vi "Set Defaults.vi"(11 "Game in":refnum<class "Game.lvclass">) -> (3 "Game out":refnum<class "Game.lvclass">)   [LabVIEW 2020, in "Conditum-Example.lvlib" / "Game.lvclass"]
uses:
  Game.lvclass
  Game.lvclass/Game.ctl
  Conditum/Columns/Entity/Entity.lvclass
  Conditum/Columns/Entity Collection/Entity Collection.lvclass
  Conditum/Columns/String/String.lvclass
  Conditum/Columns/Timestamp/Timestamp.lvclass
  Conditum/Columns/Boolean/Boolean.lvclass
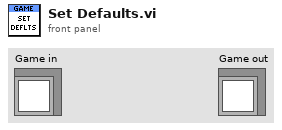
[diagram p1: front panel]
types:
  T1 = typedef "Conditum-Example.lvlib/Game.lvclass/Columns.ctl" = cluster{"Owner":refnum<class "Entity.lvclass">, "Players":refnum<class "Entity Collection.lvclass">, "Name":refnum<class "String.lvclass">, "Started":refnum<class "Timestamp.lvclass">, "Completed":refnum<class "Boolean.lvclass">}
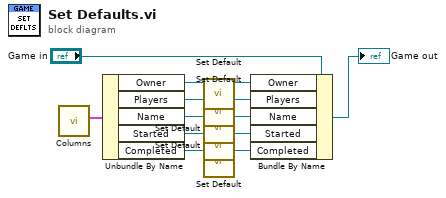
[diagram p0: block diagram]
diagram:
  n1 = call "Columns.vi"() -> ("Columns"=w13:T1)  [unwired: 11 in]
  n2 = Unbundle By Name(w13) -> ("Owner"=w12:refnum<class "Entity.lvclass">, "Players"=w10:refnum<class "Entity Collection.lvclass">, "Name"=w9:refnum<class "String.lvclass">, "Started"=w8:refnum<class "Timestamp.lvclass">, "Completed"=w11:refnum<class "Boolean.lvclass">)
  n3 = call-dynamic "Set Default.vi"("Relation in"=w12) -> ("Relation out"=w6:refnum<class "Entity.lvclass">)  [unwired: 10 in]
  n4 = call-dynamic "Set Default.vi"("Relation in"=w10) -> ("Relation out"=w1:refnum<class "Entity Collection.lvclass">)  [unwired: 10 in]
  n5 = call-dynamic "Set Default.vi"("String in"=w9) -> ("String out"=w2:refnum<class "String.lvclass">)  [unwired: 10 in]
  n6 = call-dynamic "Set Default.vi"("Timestamp in"=w8) -> ("Timestamp out"=w3:refnum<class "Timestamp.lvclass">)  [unwired: 10 in]
  n7 = call-dynamic "Set Default.vi"("Boolean in"=w11) -> ("Boolean out"=w4:refnum<class "Boolean.lvclass">)  [unwired: 10 in]
  n8 = Bundle By Name(cluster="Game in", "Owner"=w6, "Players"=w1, "Name"=w2, "Started"=w3, "Completed"=w4) -> (→"Game out":refnum<class "Game.lvclass">)
